vi "Main_03A.vi"() -> ()   [LabVIEW 2025]
uses:
  Utility/Universal Utility/TypeDefs_Utility/Cluster_Row-Column.ctl
  9e3f57c0-2ef8-4495-8287-c6a42a5fb955.vi
  Utility/Universal Utility/TypeDefs_Utility/ENUM_4 Directions U-D-L-R.ctl
  Utility/Universal Utility/TypeDefs_Utility/ENUM_8 Directions U-D-L-R.ctl
panel:
  out "max Jolts":i32[](array[numeric])
  out "MATCH":bool
  in  "Select Data":enum32{"Example", "Puzzle"}(tab)
  in  "EX Target":u32=357
  in  "Example":string="987654321111111\n811111111111119\n234234234234278\n818181911112111"
  in  "Puzzle":string="2233643232222242333443433223122333324326451323323334325223136631334332233233323164354342233332238233\n6436547659356357277564683346658554864789866767856546426667566576537557576764753366663247799566575359\n4322212422212222222222112222221252322222222222121152214312222222226122122421262632221222352222223522\n5242873574376258254526262841222235756126125363535226724625252231422222223232432416114933476433226425\n4423241233122222212222152223222321224343432221222131223143222222223442622361254132221212223321223232\n23544433354444444444454732334364434434474343434534643724444447444443414354445434434336456444466..."
  in  "Puzzle Target":u32=17074
  out "Answer":u32
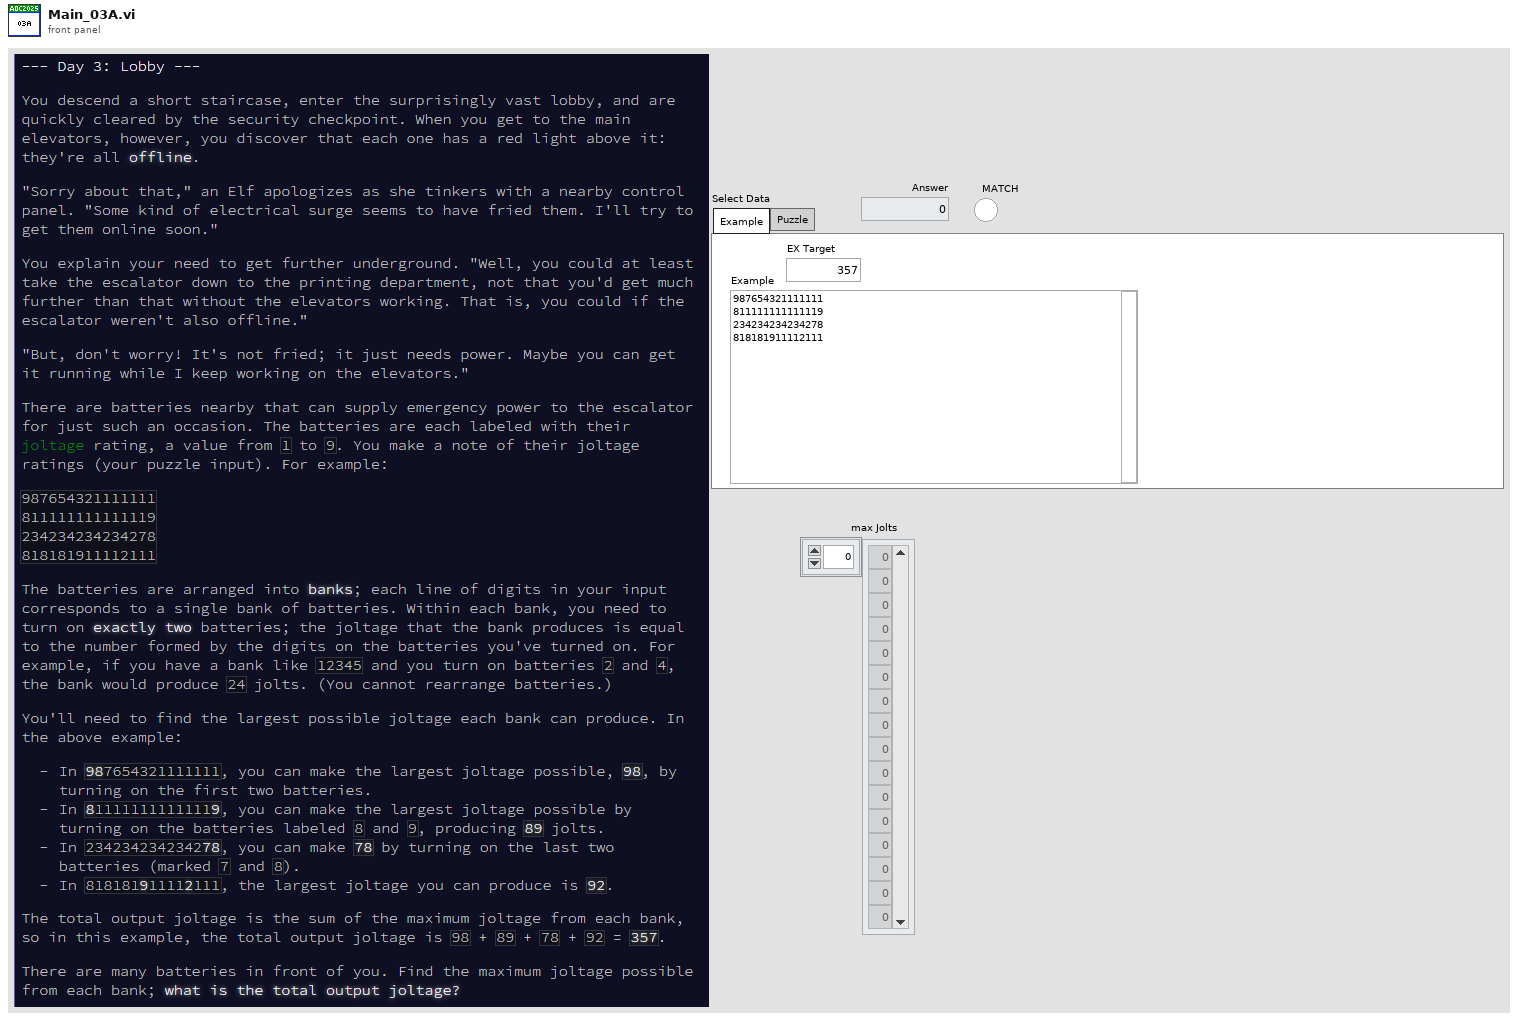
[diagram p1: front panel]
types:
  T1 = typedef "ENUM_8 Directions U-D-L-R.ctl" = enum16{"Up;-1,0", "Up-Right;-1,1", "Right;0,1", "Down-Right;1,1", "Down;1,0", "Down-Left;1,-1", "Left;0,-1", "Up-Left;-1,-1"}
  T2 = typedef "ENUM_4 Directions U-D-L-R.ctl" = enum16{"Up;-1,0", "Right;0,1", "Down;1,0", "Left;0,-1"}
  T3 = typedef "Cluster_Row-Column.ctl" = cluster{"R":i32, "C":i32}
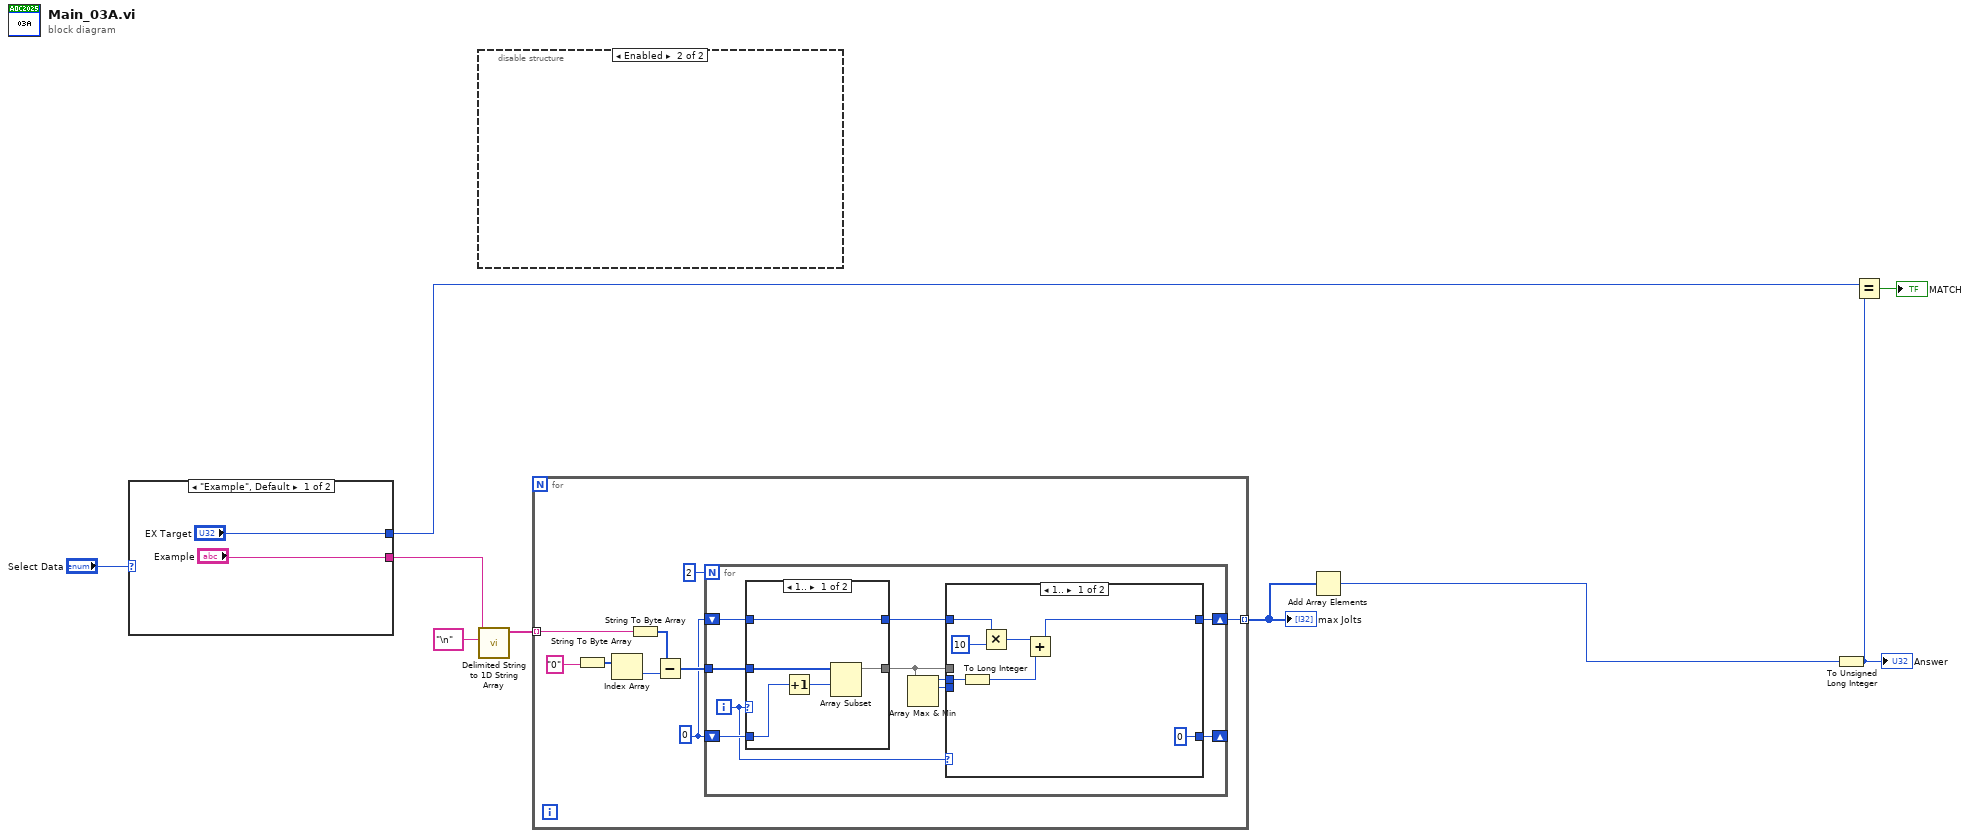
[diagram p0: block diagram]
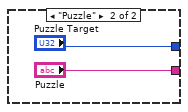
[diagram p2: hidden frame]
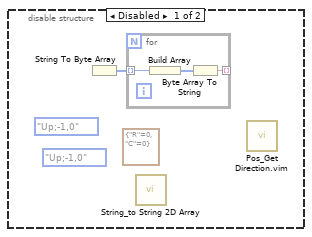
[diagram p3: hidden frame]
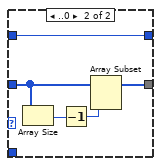
[diagram p4: hidden frame]
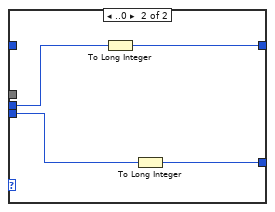
[diagram p5: hidden frame]
diagram:
  n1 = case shown="\"Example\", Default" "Select Data" {
    tunnel: ["Example" "Puzzle"] -> w7
    tunnel: ["EX Target" "Puzzle Target"] -> w3
    frame "Example", Default {
    }
    frame "Puzzle" {
    }
  }
  n2 = disable-structure shown="Enabled" {
    frame Disabled {
      (unwired) ENUM_8_Directions_U-D-L-R."Up;-1,0" ("Direction 8")
      (unwired) ENUM_4_Directions_U-D-L-R."Up;-1,0" ("Direction")
      (unwired) T3 {"R"=0, "C"=0} ("Position")
      n3 = String To Byte Array() -> (unsigned byte array=w14:u8[])  [unwired: 1 in]
      n4 = for {
        tunnel: w14 -> [w17] mode=indexing
        tunnel: [w15] -> _ mode=indexing
        n5 = Build Array(w17) -> (w16:u8[])
        n6 = Byte Array To String(unsigned byte array=w16) -> (string=w15:string)
      }
      n7 = call "String_to String 2D Array.vi"() -> ()  [unwired: 11 in, 1 out]
      n8 = call "Pos_Get Direction.vim"() -> ()  [unwired: 11 in, 1 out]
    }
    frame Enabled {
    }
  }
  n9 = call <vilib>:"Delimited String to 1D String Array.vi"("delimiter"="\n" ("delimiter (Tab)"), "delimited string"=w7) -> ("string array"=w8:string[])  [unwired: 9 in]
  n10 = for {
    tunnel: w8 -> [w22] mode=indexing
    tunnel: [w18] -> w2 mode=indexing
    w20 = 0
    n11 = String To Byte Array(string="0") -> (unsigned byte array=w24:u8[])
    n12 = Index Array(array=w24) -> (element=w25:u8)  [unwired: 1 in]
    n13 = String To Byte Array(string=w22) -> (unsigned byte array=w26:u8[])
    n14 = Subtract(x=w26, y=w25) -> (x-y=w21:u8[])
    n15 = for {
      N: 2 -> [_]
      tunnel: w21 -> [w36]
      shift-right: [w27] -> _
      shift-left: w20 -> [w34]
      shift-right: [w28] -> w18
      shift-left: w20 -> [w32]
      i -> [w33]
      n16 = case shown="1.." w33 {
        tunnel: w36 -> [w41 w46]
        tunnel: [w39 w43] -> w35
        tunnel: w34 -> [w40 _]
        tunnel: w32 -> [w37 w42]
        tunnel: [w37 w42] -> w31
        frame 1.. {
          n17 = Increment(x=w40) -> (x+1=w38:i32)
          n18 = Array Subset(array=w41, index=w38) -> (w39:u8[])  [unwired: 1 in]
        }
        frame ..0 {
          n19 = Array Size(array=w46) -> (size(s)=w45:i32)
          n20 = Decrement(x=w45) -> (x-1=w44:i32)
          n21 = Array Subset(array=w46, length=w44) -> (w43:u8[])  [unwired: 1 in]
        }
      }
      n22 = Array Max & Min(array=w35) -> (max value=w30:u8, max index (indices)=w29:i32)  [unwired: 2 out]
      n23 = case shown="1.." w33 {
        tunnel: w35 -> [_ _]
        tunnel: w31 -> [w53 _]
        tunnel: w30 -> [w50 w57]
        tunnel: w29 -> [_ w56]
        tunnel: [w49 w55] -> w28
        tunnel: [0 w54] -> w27
        frame 1.. {
          n24 = To Long Integer(number=w50) -> (32bit integer=w48:i32)
          n25 = Multiply(x=w53, y=10) -> (x*y=w51:i32)
          n26 = Add(x=w51, y=w48) -> (x+y=w49:i32)
        }
        frame ..0 {
          n27 = To Long Integer(number=w57) -> (32bit integer=w55:i32)
          n28 = To Long Integer(number=w56) -> (32bit integer=w54:i32)
        }
      }
    }
  }
  "max Jolts" <- w2
  n29 = Add Array Elements(numeric array=w2) -> (sum=w1:i32)
  n30 = To Unsigned Long Integer(number=w1) -> (unsigned 32bit integer=w5:u32)
  "Answer" <- w5
  n31 = Equal?(x=w3, y=w5) -> (x = y?=→"MATCH":bool)
